vi "CalculateDiagnosticKeyFromSeed.vi"(0 "SeedKey DLL path":path, 1 "security level":u32=1, 2 "optional parameter (OEM specific)":i8, 5 "seed":u8[](array[numeric])=[0, 0] format="%.0x", 9 "maximum key length":u32=4, 11 "error in (no error)":errorcluster, 12 "ECU variant":i8=1) -> (3 "return value":i32, 6 "key":u8[](array[numeric]) format="%.0x", 14 "key length":u32, 15 "error out":errorcluster)   [LabVIEW 2019]
doc: "Calculates <b>key</b> to unlock diagnostic sessions using the <b>SeedKey DLL (path)</b> based on a <b>seed</b> obtained from the control unit. <b>Key</b> calculation typically depends on the desired <b>security level</b> and <b>ECU variant</b>. The resulting <b>key</b> is already truncated to <b>key length</b>.\nA <b>return value</b> other than 0 indicates an error occured during the calculation.\nThe VI tries to call <i>GenerateKeyExOpt</i> and if not successful <i>GenerateKeyEx</i>.\n\nDLL calls:\n\nKEYGENALGO_API VKeyGenResultExOpt GenerateKeyExOpt(\n const unsigned char* ipSeedArray, // Array for the seed [in]\n unsigned int iSeedArraySize, // Length of the array for the seed [in]\n const unsigned int iSecurityLevel, // Security level [in]\n const char* ipVariant, // Name of the active variant [in]\n const char* ipOptions, // Optional parameter which might be used for OEM specific information [in]\n unsigned char* iopKeyArray, // Array for the key [in, out]\n unsigned int iMaxKeyArraySize, // Maximum length of the array for the key [in]\n unsigned int& oActualKeyArraySize) // Length of the key [out]\n\nKEYGENALGO_API VKeyGenResultEx GenerateKeyEx(\n const unsigned char* iSeedArray, /* Array for the seed [in] */\n unsigned int iSeedArraySize, /* Length of the array for the seed [in] */\n const unsigned int iSecurityLevel, /* Security level [in] */\n const char* iVariant, /* Name of the active variant [in] */\n unsigned char* ioKeyArray, /* Array for the key [in, out] */\n unsigned int iKeyArraySize, /* Maximum length of the array for the key [in] */\n unsigned int& oSize /* Length of the key [out] */\n )"
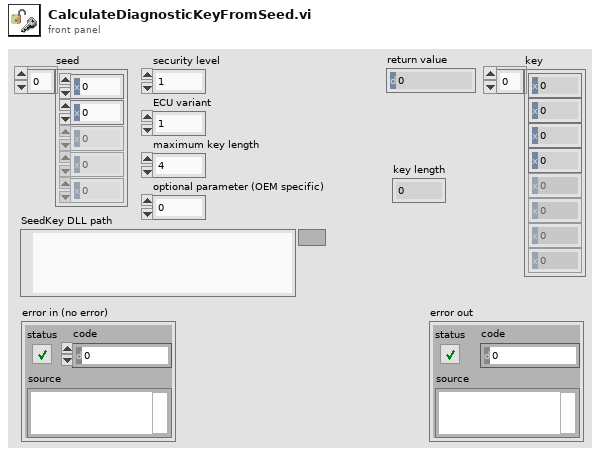
[diagram p1: front panel]
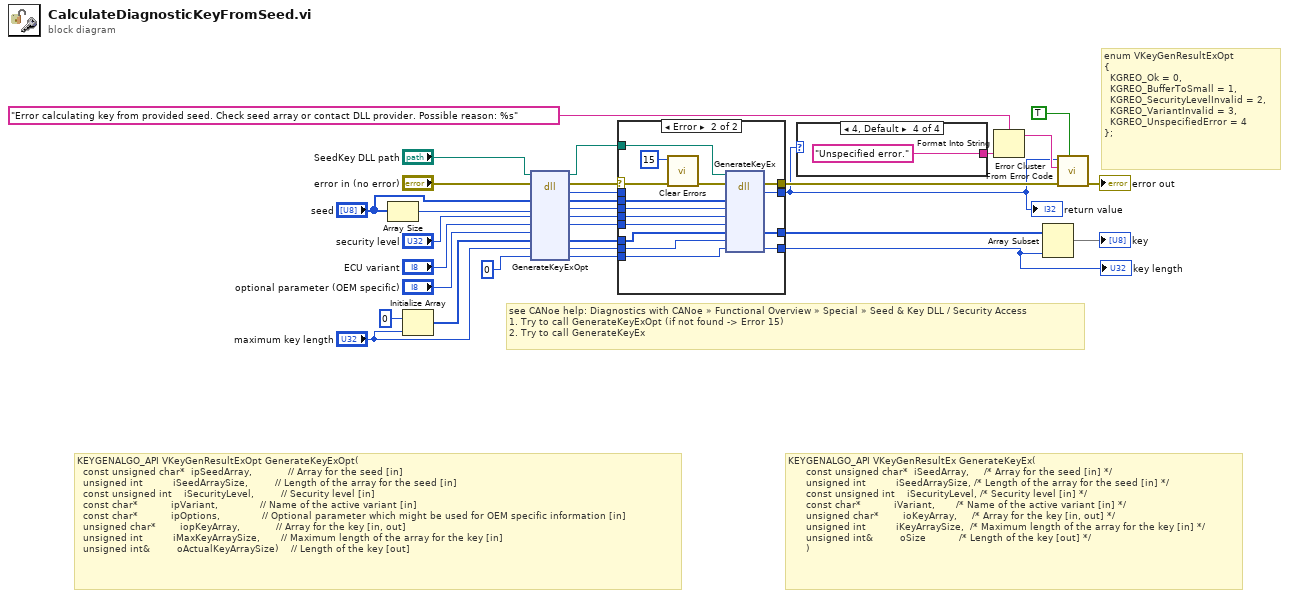
[diagram p0: block diagram]
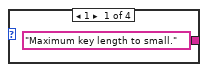
[diagram p2: hidden frame]
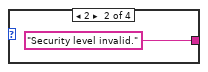
[diagram p3: hidden frame]
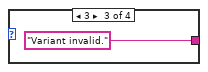
[diagram p4: hidden frame]
diagram:
  # "enum VKeyGenResultExOpt\n{\n  KGREO_Ok = 0,\n  KGREO_BufferToSmall = 1,\n  KGREO_SecurityLevelInvalid = 2,\n  KGREO_VariantInvalid = 3,\n  KGREO_UnspecifiedError = 4\n};"
  # "see CANoe help: Diagnostics with CANoe » Functional Overview » Special » Seed & Key DLL / Security Access\n1. Try to call GenerateKeyExOpt (if not found -> Error 15)\n2. Try to call GenerateKeyEx"
  # "KEYGENALGO_API VKeyGenResultExOpt GenerateKeyExOpt(\n  const unsigned char*  ipSeedArray,            // Array for the seed [in]\n  unsigned int          iSeedArraySize,         // Length of the array for the seed [in]\n  const unsigned int    iSecurityLevel,         // Security level [in]\n  const char*           ipVariant,              // Name of the active variant [in]\n  const char*           ipOptions,              // Optional parameter which might be used for OEM specific information [in]\n  unsigned char*        iopKeyArray,            // Array for the key [in, out]\n  unsigned int          iMaxKeyArraySize,       // Maximum length of the array for the key [in]\n  unsigned int&         oActualKeyArraySize)    // Length of the key [out]"
  # "KEYGENALGO_API VKeyGenResultEx GenerateKeyEx(\n      const unsigned char*  iSeedArray,     /* Array for the seed [in] */\n      unsigned int          iSeedArraySize, /* Length of the array for the seed [in] */\n      const unsigned int    iSecurityLevel, /* Security level [in] */\n      const char*           iVariant,       /* Name of the active variant [in] */\n      unsigned char*        ioKeyArray,     /* Array for the key [in, out] */\n      unsigned int          iKeyArraySize,  /* Maximum length of the array for the key [in] */\n      unsigned int&         oSize           /* Length of the key [out] */\n      )"
  n1 = Array Size(array="seed") -> (size(s)=w19:i32)
  n2 = Initialize Array(u8 0 ("element"), "maximum key length") -> (w15:u8[])
  n3 = dll-call lib="GenerateKeyExOpt.dll" fn="GenerateKeyExOpt"(path in="SeedKey DLL path", error in="error in (no error)", "iSeedArray"="seed", "iSeedArraySize"=w19, "iSecurityLevel"="security level", "iVariant"="ECU variant", "ipOptions"="optional parameter (OEM specific)", "ioKeyArray"=w15, "iKeyArraySize"="maximum key length", "oSize"=u32 0) -> (path out=w22:path, error out=w21:errorcluster, "VKeyGenResultEx"=w12:i32, "iSeedArray"=w9:u8[], "iSeedArraySize"=w8:u32, "iSecurityLevel"=w7:u32, "iVariant"=w6:i8, "ioKeyArray"=w11:u8[], "iKeyArraySize"=w5:u32, "oSize"=w10:u32)  [unwired: 2 in]
  n4 = case shown="Error" w21 {
    selector: w21 -> [w35 w43]
    tunnel: [w35 w50] -> w29
    tunnel: [w34 w49] -> w2
    tunnel: [w33 w48] -> w27
    tunnel: [w32 w47] -> w26
    tunnel: w22 -> [_ w44]
    tunnel: w12 -> [w34 _]
    tunnel: w11 -> [w33 w38]
    tunnel: w10 -> [w32 w36]
    tunnel: w9 -> [_ w42]
    tunnel: w8 -> [_ w41]
    tunnel: w7 -> [_ w40]
    tunnel: w6 -> [_ w39]
    tunnel: w5 -> [_ w37]
    frame No Error {
    }
    frame Error {
      n5 = call <vilib>:"Clear Errors.vi"("error in (no error)"=w43, "specific error code to clear (0: all)"=15) -> ("error out"=w46:errorcluster)  [unwired: 4 in, 1 out]
      n6 = dll-call lib="key_generator_extended_session.dll" fn="GenerateKeyEx"(path in=w44, error in=w46, "iSeedArray"=w42, "iSeedArraySize"=w41, "iSecurityLevel"=w40, "iVariant"=w39, "ioKeyArray"=w38, "iKeyArraySize"=w37, "oSize"=w36) -> (error out=w50:errorcluster, "VKeyGenResultEx"=w49:i32, "ioKeyArray"=w48:u8[], "oSize"=w47:u32)  [unwired: 6 in, 1 out]
    }
  }
  "key length" <- w26
  "return value" <- w2
  n7 = case shown="4, Default" w2 {
    tunnel: ["Maximum key length to small." "Security level invalid." "Variant invalid." "Unspecified error."] -> w1
    frame 1 {
    }
    frame 2 {
    }
    frame 3 {
    }
    frame 4, Default {
    }
  }
  n8 = Format Into String(format string="Error calculating key from provided seed. Check seed array or contact DLL provider. Possible reason: %s" ("error message (\"\")"), w1) -> (resulting string=w3:string)  [unwired: 2 in, 1 out]
  n9 = Array Subset(array=w27, length=w26) -> (→"key":u8[])  [unwired: 1 in]
  n10 = call <vilib>:"Error Cluster From Error Code.vi"("show call chain? (False)"=TRUE, "error in (no error)"=w29, "error message (\"\")"=w3, "error code (0)"=w2) -> ("error out"=→"error out":errorcluster)  [unwired: 5 in]
